vi "AssertSubpanelExecStateBad_Tests.vi"(11 "error in":errorcluster) -> (15 "error out":errorcluster)   [LabVIEW 2016, in "DronaTest.lvlib"]
uses:
  DronaTest.lvlib
  APIs/Stimulus/ControlValue/ValueSignalByPathString.vi
  APIs/Assert/AssertControlValue/Controls/Subpanel/AssertSubpanelVIExecBad.vi
  <vilib>/addons/_JKI Toolkits/Caraya/classes/Test/Test.lvclass
  Drona.lvlib
  APIs/Stimulus/ControlValue/ControlValue.lvlib
  APIs/Assert/AssertControlValue/Controls/Subpanel/AssertSubpanel.lvlib
  <vilib>/addons/_JKI Toolkits/Caraya/classes/Assert/Assert.lvclass
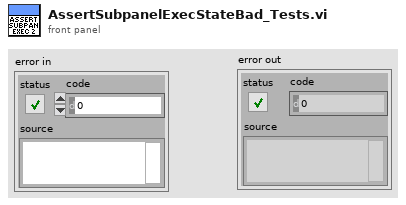
[diagram p1: front panel]
types:
  T1 = enum32{"Bad", "Idle", "Run top level", "Running"}
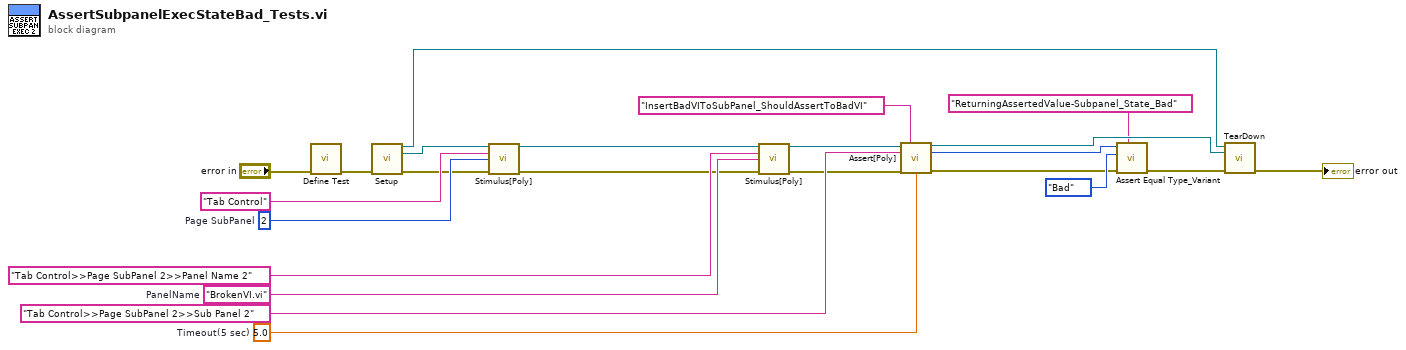
[diagram p0: block diagram]
diagram:
  w13 = 2  # Page SubPanel
  w18 = "BrokenVI.vi"  # PanelName
  w19 = 5.0  # Timeout(5 sec)
  n1 = call <vilib>:"Define Test.vi"("error in (no error)"="error in") -> ("error out"=w15:errorcluster)  [unwired: 9 in, 1 out]
  n2 = call "Setup.vi"("error in (no error)"=w15) -> ("Application Ref"=w7:refnum<vi>, "VI out"=w6:refnum<vi>, "error out"=w10:errorcluster)  [unwired: 12 in]
  n3 = call-poly "Stimulus[Poly].vi"("VI Reference In"=w6, "Control Path"="Tab Control", "Value (Signaling)"=w13, "error in"=w10) -> ("VI Reference Out"=w16:refnum<vi>, "error out"=w12:errorcluster)  [unwired: 10 in]
  n4 = call-poly "Stimulus[Poly].vi"("VI Reference In"=w16, "Control Path"="Tab Control>>Page SubPanel 2>>Panel Name 2", "Value (Signaling)"=w18, "error in"=w12) -> ("VI Reference Out"=w11:refnum<vi>, "error out"=w17:errorcluster)  [unwired: 10 in]
  n5 = call-poly "Assert[Poly].vi"("VI Reference In"=w11, "Test Label"="InsertBadVIToSubPanel_ShouldAssertToBadVI" ("Label"), "Control Path"="Tab Control>>Page SubPanel 2>>Sub Panel 2", "Error In"=w17, "Timeout(5 sec)"=w19) -> ("VI Reference Out"=w8:refnum<vi>, "Asserted Value"=w1:T1, "Error Out"=w4:errorcluster)  [unwired: 8 in]
  n6 = call <vilib>:"Assert Equal Type_Variant.vi"("Label"="ReturningAssertedValue-Subpanel_State_Bad", "error in (no error)"=w4, "Y"=T1."Bad" ("Asserted Value"), "X"=w1) -> ("error out"=w3:errorcluster)  [unwired: 6 in, 1 out]
  n7 = call "TearDown.vi"("Application Ref"=w7, "VI in"=w8, "error in (no error)"=w3) -> ("error out"=→"error out":errorcluster)  [unwired: 12 in]
